vi "Write Customer Name.vi"(10 "Customer Name":string, 11 "Beverage in":refnum<class "Beverage.lvclass">) -> (3 "Beverage in 2":refnum<class "Beverage.lvclass">)   [LabVIEW 2013, in "Beverage.lvclass"]
uses:
  Beverage.lvclass
  Beverage.lvclass/Beverage.ctl
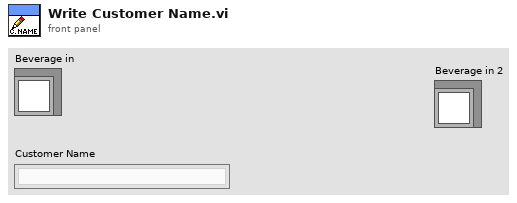
[diagram p1: front panel]
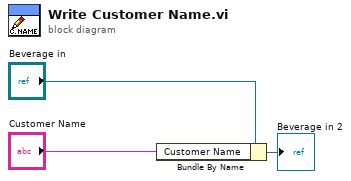
[diagram p0: block diagram]
diagram:
  n1 = Bundle By Name(cluster="Beverage in", "Customer Name"="Customer Name") -> (→"Beverage in 2":refnum<class "Beverage.lvclass">)
